vi "Configure Trigger Source.vi"(8 "error in (no error)":errorcluster, 9 "External Level":dbl, 10 "Trigger Source":enum16{"Immediate", "External"}(ring), 11 "SA-FSW in":refnum<class "SA-FSW.lvclass">) -> (0 "error out":errorcluster, 3 "SA-FSW out":refnum<class "SA-FSW.lvclass">)   [LabVIEW 2020, in "SA-FSW.lvclass"]
uses:
  SA-FSW.lvclass
  C:/Sandbox/Git_Sandbox/WiSpry Test Framework source code (LV20)/WiSpry Test Framework/Instruments/Instrument.lvclass
  Instrument.lvclass/Instrument.ctl
  Instrument.lvclass
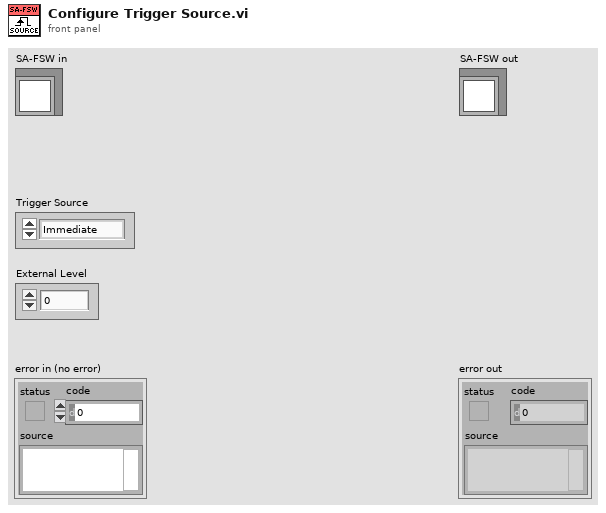
[diagram p1: front panel]
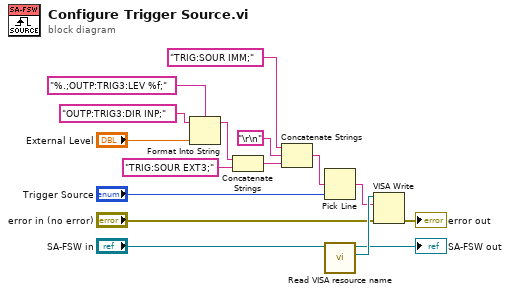
[diagram p0: block diagram]
diagram:
  n1 = Format Into String(format string="%.;OUTP:TRIG3:LEV %f;", initial string="OUTP:TRIG3:DIR INP;", "External Level") -> (resulting string=w12:string)  [unwired: 1 in, 1 out]
  n2 = Concatenate Strings(w12, "TRIG:SOUR EXT3;" ("string")) -> (w10:string)
  n3 = Concatenate Strings("TRIG:SOUR IMM;", "\r\n", w10) -> (w7:string)
  n4 = Pick Line(multi-line string=w7, line index="Trigger Source") -> (output string=w4:string)  [unwired: 1 in]
  n5 = call "Read VISA resource name.vi"("Instrument in"="SA-FSW in") -> ("VISA resource name"=w5:refnum<visa-resource-name>, "Instrument out"=→"SA-FSW out":refnum<class "SA-FSW.lvclass">)  [unwired: 9 in]
  n6 = VISA Write(VISA resource name=w5, write buffer=w4, error in (no error)="error in (no error)") -> (error out=→"error out":errorcluster)  [unwired: 2 out]
